vi "Prober_ChuckUpDown.vi"(8 "error in (no error)":errorcluster, 10 "Direction":enum16{"up", "down"}(ring), 11 "ProbeStationControl in":refnum<class "ProbeStationControl.lvclass">) -> (0 "error out":errorcluster, 2 "Chuck at CONTACT?":bool=TRUE, 3 "ProbeStationControl out":refnum<class "ProbeStationControl.lvclass">)   [LabVIEW 2018, in "ProbeStationControl.lvclass"]
uses:
  ProbeStationControl.lvclass
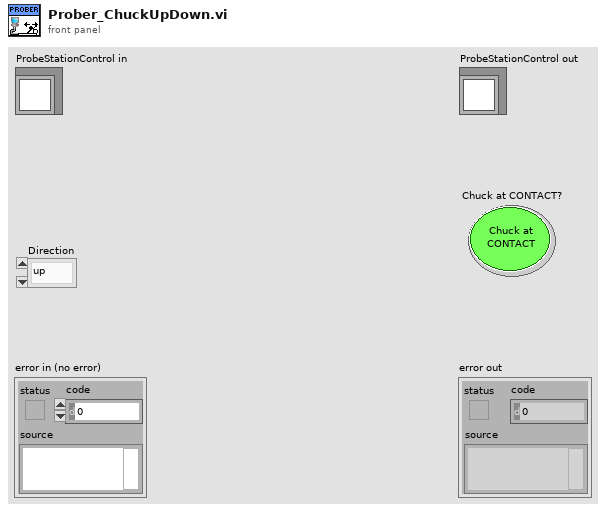
[diagram p1: front panel]
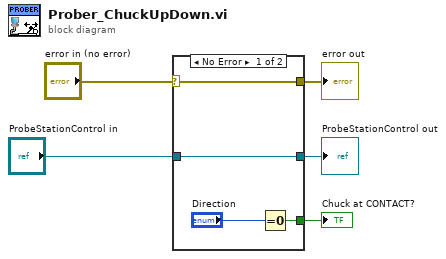
[diagram p0: block diagram]
diagram:
  n1 = case shown="No Error" "error in (no error)" {
    selector: "error in (no error)" -> [w6 w11]
    tunnel: [w6 w11] -> w4
    tunnel: "ProbeStationControl in" -> [w7 w10]
    tunnel: [w8 _] -> w3
    tunnel: [w7 w10] -> w1
    frame No Error {
      n2 = Equal To 0?(x="Direction") -> (x = 0?=w8:bool)
    }
    frame Error {
    }
  }
  "error out" <- w4
  "Chuck at CONTACT?" <- w3
  "ProbeStationControl out" <- w1
